vi "Disconnect.vi"(8 "error in":errorcluster, 11 "57XX in":refnum<class "57XX.lvclass">) -> (0 "error out":errorcluster, 3 "57XX out":refnum<class "57XX.lvclass">)   [LabVIEW 2019, in "57XX.lvlib" / "57XX.lvclass"]
uses:
  Library/57XX.lvclass
  Library/57XX.lvclass/57XX.ctl
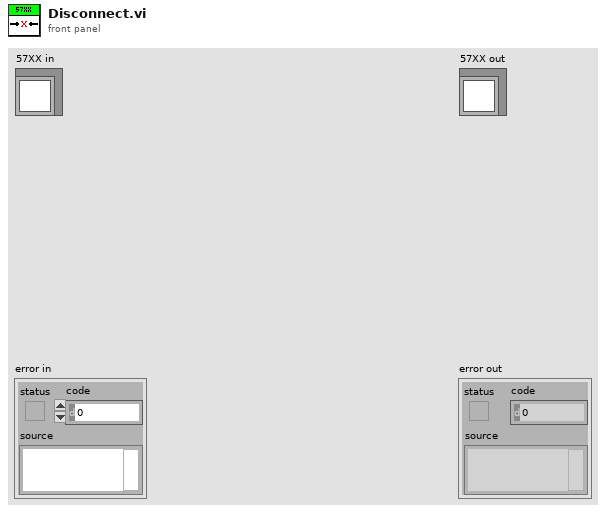
[diagram p1: front panel]
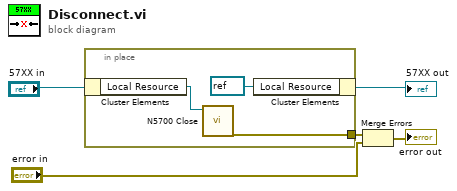
[diagram p0: block diagram]
diagram:
  n1 = in-place {
    in-place-border: [w6] -> w2
    n2 = in-place-cluster #1("57XX in") -> ("Local Resource"=w8:refnum<visa-resource-name>)
    n3 = call <instrlib>:"N5700 Close.vi"("VISA name"=w8) -> ("error out"=w6:errorcluster)  [unwired: 7 in]
    n4 = in-place-cluster #1("Local Resource"=refnum<visa-resource-name> refnum) -> (→"57XX out":refnum<class "57XX.lvclass">)
  }
  n5 = Merge Errors(w2, "error in") -> (→"error out":errorcluster)
